vi "playback_choose_freq.vi"() -> ()   [LabVIEW 2012]
doc: "This VI will initialize the FPGA VI and read a user-defined number of samples from a DMA FIFO. When the data acquisition is complete this VI will read status information from the FPGA VI.\n\nFollow these instructions to run the VI.\n\n1. Select your RIO device from the dropdown.\n2. Set the sample period, number of samples to acquire per channel, and DMA block read size. \n\nNote: the block read size should be set to balance load on the host processor and the update rate of the user interface. A small block read size will update the user interface more often but will result in a higher load on the host processor."
uses:
  <vilib>/Analysis/3filter.llb/Filter Passband Type.ctl
  <vilib>/Analysis/3filter.llb/Elliptic Filter (DBL).vi
  <vilib>/Analysis/3filter.llb/Butterworth Filter (DBL).vi
  <vilib>/Analysis/NI_AALBase.lvlib
panel:
  in  "Noise length":i32=50
  out "threshold 0":dbl(graph)
  in  "Filter mode":enum16{"Elliptic", "Butterworth"}(ring)=enum."Butterworth"
  in  "order":i32=3
  in  "low cutoff freq: fl":dbl=20000.0
  in  "high cutoff freq: fh":dbl=30000.0
  out "Selected Index":i32
  out "Ratio at Index (%)":dbl
  in  "Threshold":dbl=0.1
  out "Index 0":dbl
  out "Index 1":dbl
  out "Index 2":dbl
  out "Index 3":dbl
  in  "noise min":dbl=0.001
  out "amplitude 0":dbl
  out "amplitude 1":dbl
  out "amplitude 2":dbl
  out "amplitude 3":dbl
  in  "Portion Duration":i32=600
  in  "Altitude":dbl=2.0
  out "x":dbl format="%#_6f"
  out "y":dbl format="%#_6f"
  out "z":dbl
  out "yaw":dbl
  out "pitch":dbl
  out "Yaw Chart":dbl(graph)
  in  "Mode":T1(ring)=enum."Use Far Field"
  out "Threshold 0":dbl
  out "Threshold 1":dbl
  out "Threshold 2":dbl
  out "Threshold 3":dbl
  in  "threshold ratio":dbl=3.0
  out "bad signal?":bool
  out "ROS  Error":bool
  in  "Send to ROS":bool
  out "dt1":dbl
  out "dt2":dbl
  out "dt3":dbl
  out "Forward":dbl
  out "Sidemove":dbl
  out "Extracted signal":dbl[][](graph)
  in  "Select Frequency":dbl=24000.0
  out "frequency 2":dbl
  out "frequency 1":dbl
  out "Chosen Signal":dbl[][](graph)
  in  "Wait?":bool
  in  "Next Signal":bool
  in  "Filename":path=path "D:/Recorded/US Test/Robosub day 1/pinger_in_front.tdms"
  out "Original Filtered Ch0":dbl[](graph)
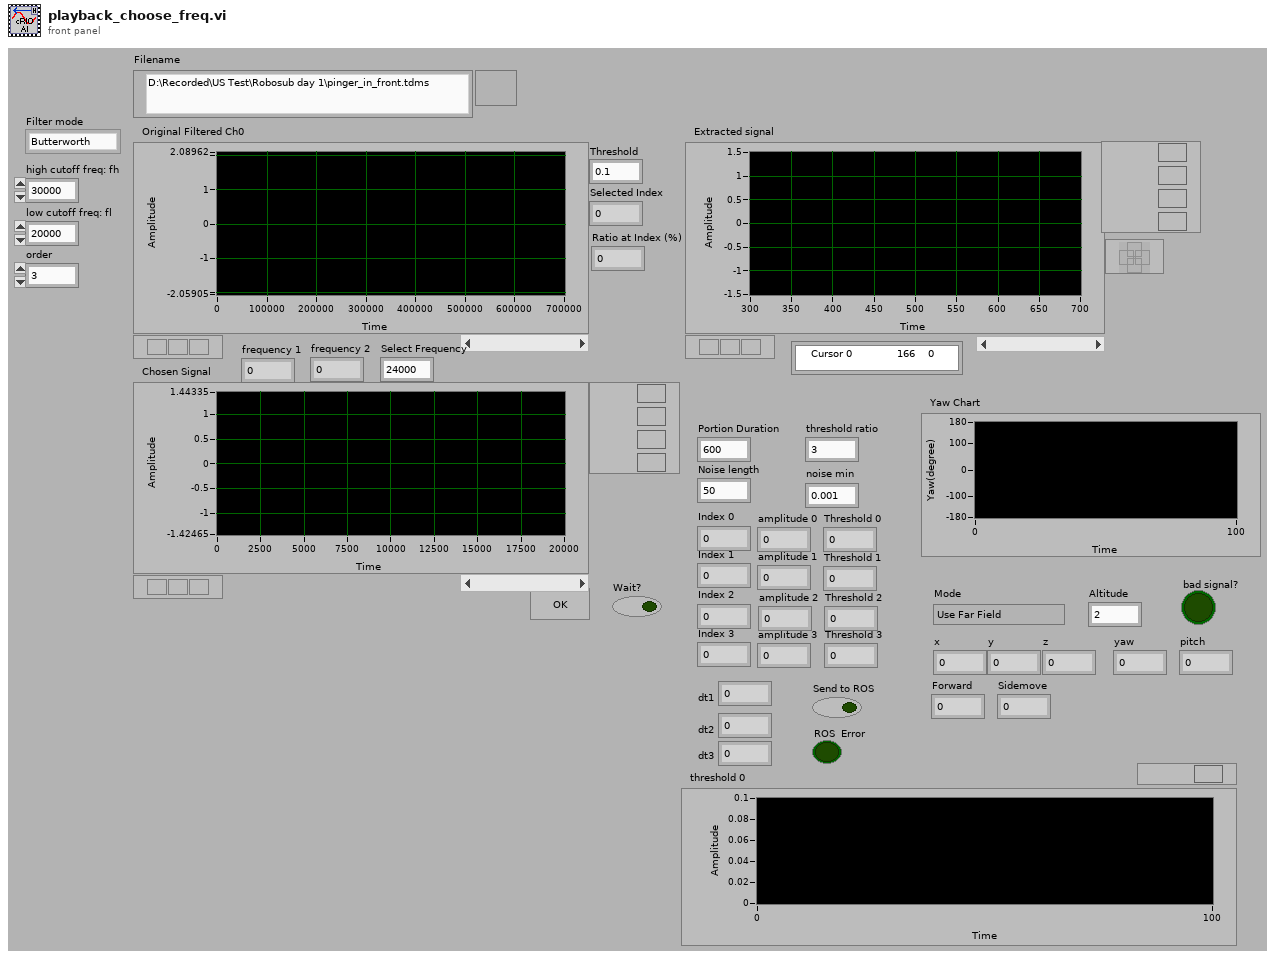
[diagram p1: front panel]
types:
  T1 = enum16{"Use Near Field", "Use Far Field", "Far Field with 3 hydrophones"}
  T2 = typedef "NI_AALBase.lvlib/Filter Passband Type.ctl" = enum32{"Lowpass", "Highpass", "Bandpass", "Bandstop"}
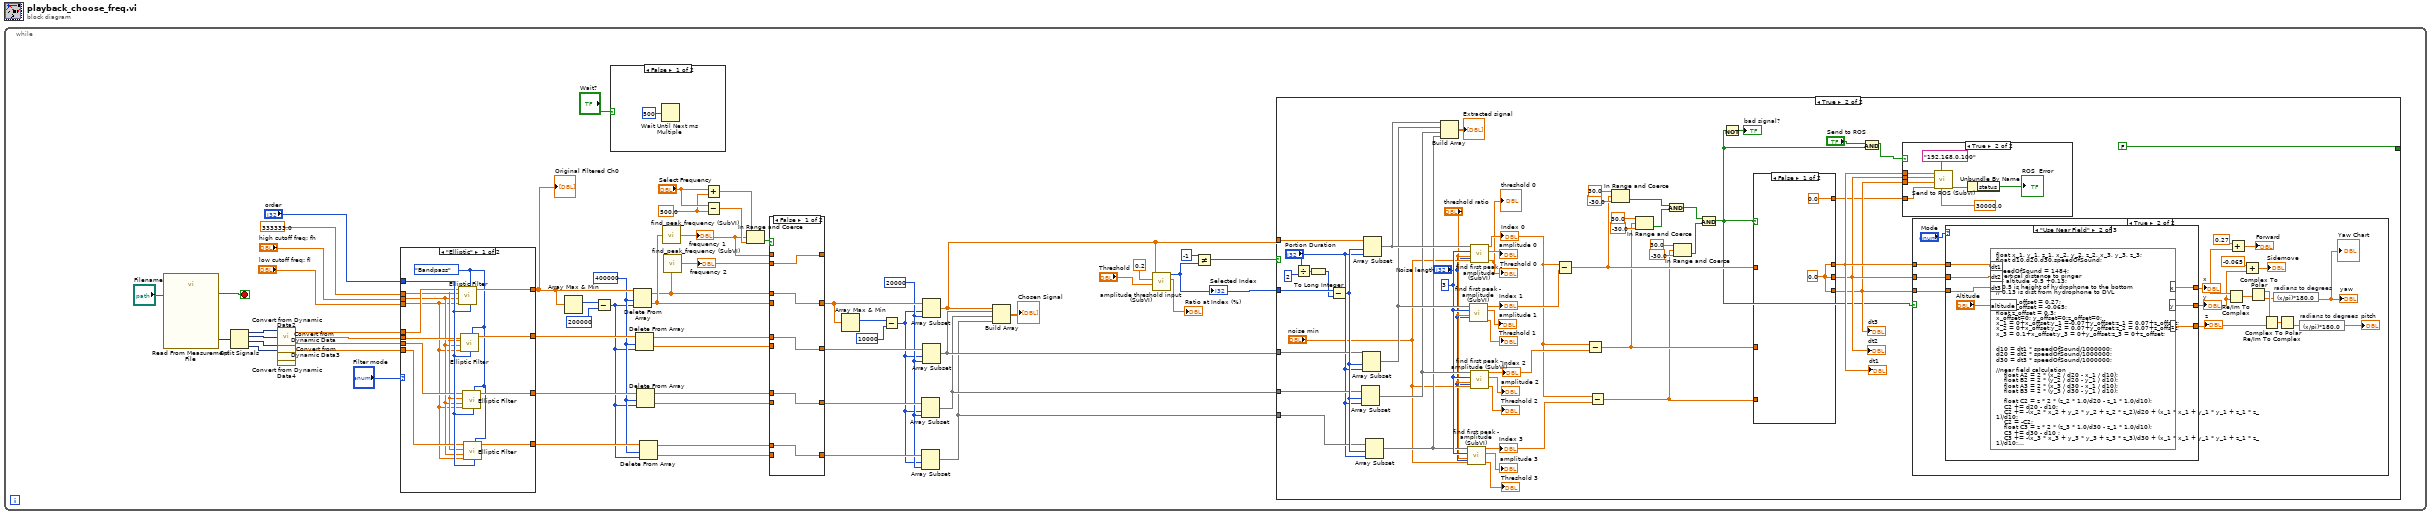
[diagram p0: block diagram]
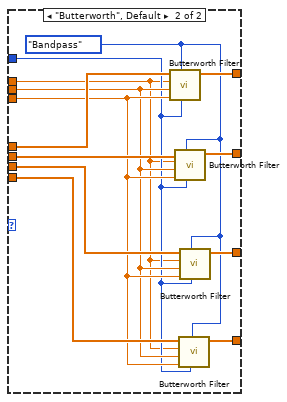
[diagram p2: hidden frame]
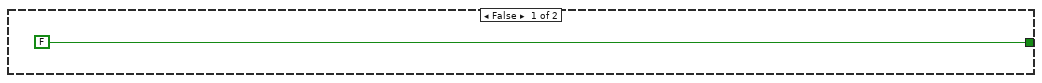
[diagram p3: hidden frame]
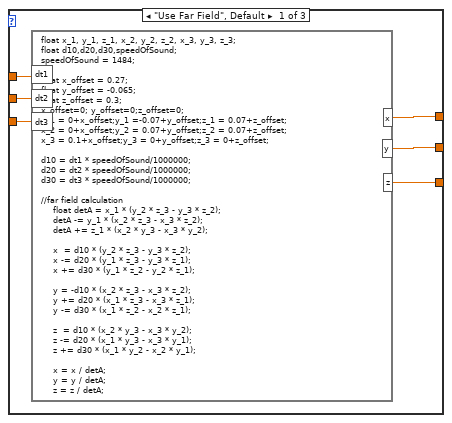
[diagram p5: hidden frame]
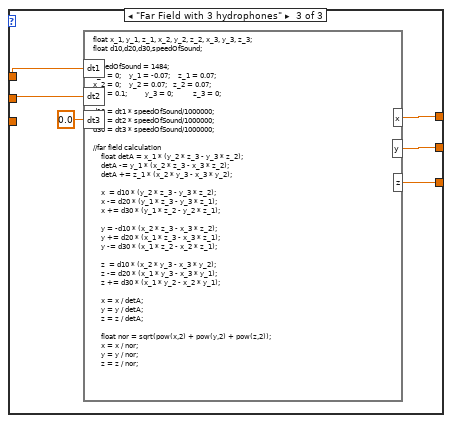
[diagram p6: hidden frame]
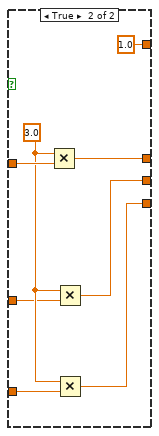
[diagram p8: hidden frame]
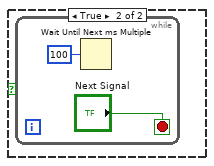
[diagram p9: hidden frame]
diagram:
  n1 = while {
    stop <- w52 stop-if-true
    w23 = 500.0 ("y")
    w29 = 20000 ("length")
    w43 = 400000 ("Portion Duration")
    n2 = call "Read From Measurement File"("Filename"="Filename") -> ("Signals"=w56:dynamicdata, "EOF?"=w52:bool)  [unwired: 5 in, 4 out]
    n3 = Split Signals(w56) -> (w3:dynamicdata, w59:dynamicdata, w58:dynamicdata, w57:dynamicdata)  [unwired: 4 in]
    n4 = call "Convert from Dynamic Data"("Dynamic Data Type"=w3) -> ("Array"=w50:dbl[])  [unwired: 3 in]
    n5 = call "Convert from Dynamic Data2"("Dynamic Data Type"=w59) -> ("Array"=w55:dbl[])  [unwired: 3 in]
    n6 = call "Convert from Dynamic Data3"("Dynamic Data Type"=w58) -> ("Array"=w53:dbl[])  [unwired: 3 in]
    n7 = call "Convert from Dynamic Data4"("Dynamic Data Type"=w57) -> ("Array"=w54:dbl[])  [unwired: 3 in]
    n8 = case shown="\"Elliptic\"" "Filter mode" {
      tunnel: w55 -> [w66 w85]
      tunnel: w54 -> [w64 w84]
      tunnel: w53 -> [w65 w83]
      tunnel: w50 -> [w67 w82]
      tunnel: [w72 w81] -> w49
      tunnel: [w71 w80] -> w46
      tunnel: [w70 w79] -> w45
      tunnel: [w69 w78] -> w44
      tunnel: "low cutoff freq: fl" -> [w60 w77]
      tunnel: "high cutoff freq: fh" -> [w61 w76]
      tunnel: "order" -> [w68 w75]
      tunnel: 333333.0 ("sampling freq: fs") -> [w62 w74]
      frame "Elliptic" {
        w63 = Filter_Passband_Type."Bandpass" ("filter type")
        n9 = call-poly <vilib>:"Elliptic Filter.vi"("order"=w68, "filter type"=w63, "low cutoff freq: fl"=w60, "high cutoff freq: fh"=w61, "sampling freq: fs"=w62, "X"=w67) -> ("Filtered X"=w72:dbl[])  [unwired: 4 in, 1 out]
        n10 = call-poly <vilib>:"Elliptic Filter.vi"("order"=w68, "filter type"=w63, "low cutoff freq: fl"=w60, "high cutoff freq: fh"=w61, "sampling freq: fs"=w62, "X"=w66) -> ("Filtered X"=w71:dbl[])  [unwired: 4 in, 1 out]
        n11 = call-poly <vilib>:"Elliptic Filter.vi"("order"=w68, "filter type"=w63, "low cutoff freq: fl"=w60, "high cutoff freq: fh"=w61, "sampling freq: fs"=w62, "X"=w65) -> ("Filtered X"=w70:dbl[])  [unwired: 4 in, 1 out]
        n12 = call-poly <vilib>:"Elliptic Filter.vi"("order"=w68, "filter type"=w63, "low cutoff freq: fl"=w60, "high cutoff freq: fh"=w61, "sampling freq: fs"=w62, "X"=w64) -> ("Filtered X"=w69:dbl[])  [unwired: 4 in, 1 out]
      }
      frame "Butterworth", Default {
        w73 = Filter_Passband_Type."Bandpass" ("filter type")
        n13 = call-poly <vilib>:"Butterworth Filter.vi"("order"=w75, "filter type"=w73, "low cutoff freq: fl"=w77, "high cutoff freq: fh"=w76, "sampling freq: fs"=w74, "X"=w82) -> ("Filtered X"=w81:dbl[])  [unwired: 2 in, 1 out]
        n14 = call-poly <vilib>:"Butterworth Filter.vi"("order"=w75, "filter type"=w73, "low cutoff freq: fl"=w77, "high cutoff freq: fh"=w76, "sampling freq: fs"=w74, "X"=w85) -> ("Filtered X"=w80:dbl[])  [unwired: 2 in, 1 out]
        n15 = call-poly <vilib>:"Butterworth Filter.vi"("order"=w75, "filter type"=w73, "low cutoff freq: fl"=w77, "high cutoff freq: fh"=w76, "sampling freq: fs"=w74, "X"=w84) -> ("Filtered X"=w78:dbl[])  [unwired: 2 in, 1 out]
        n16 = call-poly <vilib>:"Butterworth Filter.vi"("order"=w75, "filter type"=w73, "low cutoff freq: fl"=w77, "high cutoff freq: fh"=w76, "sampling freq: fs"=w74, "X"=w83) -> ("Filtered X"=w79:dbl[])  [unwired: 2 in, 1 out]
      }
    }
    "Original Filtered Ch0" <- w49
    n17 = Array Max & Min(array=w49) -> (max index (indices)=w48:i32)  [unwired: 3 out]
    n18 = Subtract(x=w48, y=200000) -> (x-y=w42:i32)
    n19 = case shown="False" "Wait?" {
      frame False {
        n20 = Wait Until Next ms Multiple(millisecond multiple=u32 500) -> ()  [unwired: 1 out]
      }
      frame True {
        n21 = while {
          stop <- "Next Signal" stop-if-true
          n22 = Wait Until Next ms Multiple(millisecond multiple=u32 100) -> ()  [unwired: 1 out]
        }
      }
    }
    n23 = Delete From Array(array=w49, length=w43, index=w42) -> (deleted portion=w26:dbl[], array with subset deleted=w25:dbl[])
    n24 = Delete From Array(array=w46, length=w43, index=w42) -> (deleted portion=w41:dbl[], array with subset deleted=w38:dbl[])
    n25 = Delete From Array(array=w45, length=w43, index=w42) -> (deleted portion=w40:dbl[], array with subset deleted=w37:dbl[])
    n26 = Delete From Array(array=w44, length=w43, index=w42) -> (deleted portion=w39:dbl[], array with subset deleted=w36:dbl[])
    n27 = call "find_peak_frequency (SubVI).vi"("Signal"=w26) -> ("Frequency"=w19:dbl)
    "frequency 1" <- w19
    n28 = call "find_peak_frequency (SubVI).vi"("Signal"=w25) -> ("Frequency"=w18:dbl)
    "frequency 2" <- w18
    n29 = Add(x="Select Frequency", y=w23) -> (x+y=w21:dbl)
    n30 = Subtract(x="Select Frequency", y=w23) -> (x-y=w20:dbl)
    n31 = In Range and Coerce(upper limit=w21, x=w19, lower limit=w20) -> (In Range?=w22:bool)  [unwired: 1 out]
    n32 = case shown="False" w22 {
      tunnel: w26 -> [_ w207]
      tunnel: w41 -> [_ w206]
      tunnel: w40 -> [_ w205]
      tunnel: w39 -> [_ w204]
      tunnel: w25 -> [w202 _]
      tunnel: w38 -> [w201 _]
      tunnel: w37 -> [w200 _]
      tunnel: w36 -> [w199 _]
      tunnel: [w202 w207] -> w33
      tunnel: [w201 w206] -> w32
      tunnel: [w200 w205] -> w31
      tunnel: [w199 w204] -> w30
      tunnel: [w198 w203] -> _
      tunnel: w19 -> [_ w203]
      tunnel: w18 -> [w198 _]
      frame False {
      }
      frame True {
      }
    }
    n33 = Array Max & Min(array=w33) -> (max index (indices)=w34:i32)  [unwired: 3 out]
    n34 = Subtract(x=w34, y=10000) -> (x-y=w28:i32)
    n35 = Array Subset(array=w31, index=w28, length=w29) -> (w8:dbl[])
    n36 = Array Subset(array=w30, index=w28, length=w29) -> (w7:dbl[])
    n37 = Array Subset(array=w33, index=w28, length=w29) -> (w10:dbl[])
    n38 = Array Subset(array=w32, index=w28, length=w29) -> (w9:dbl[])
    n39 = Build Array(w10, w9, w8, w7) -> (→"Chosen Signal":dbl[][])
    n40 = call "amplitude threshold input (SubVI).vi"("threshold"="Threshold", "%max amplitude"=0.2, "Array"=w10) -> ("actual ratio (%)"=→"Ratio at Index (%)":dbl, "Index"=w11:i32)  [unwired: 7 in]
    "Selected Index" <- w11
    n41 = Not Equal?(x=-1 ("y"), y=w11) -> (x != y?=w15:bool)
    n42 = case shown="True" w15 {
      tunnel: w9 -> [_ w138]
      tunnel: w8 -> [_ w137]
      tunnel: w7 -> [_ w136]
      tunnel: w10 -> [_ w135]
      tunnel: w11 -> [_ w134]
      tunnel: [FALSE ("Debug") FALSE ("Debug")] -> _
      frame False {
      }
      frame True {
        w100 = 3
        n43 = Divide(x="Portion Duration", y=2) -> (x/y=w131:dbl)
        n44 = To Long Integer(number=w131) -> (32bit integer=w130:i32)
        n45 = Subtract(x=w134, y=w130) -> (x-y=w139:i32)
        n46 = Array Subset(array=w137, index=w139, length="Portion Duration") -> (w101:dbl[])
        n47 = Array Subset(array=w138, index=w139, length="Portion Duration") -> (w105:dbl[])
        n48 = Array Subset(array=w135, index=w139, length="Portion Duration") -> (w107:dbl[])
        n49 = Array Subset(array=w136, index=w139, length="Portion Duration") -> (w99:dbl[])
        n50 = Build Array(w107, w105, w101, w99) -> (→"Extracted signal":dbl[][])
        n51 = call "find first peak - amplitude (SubVI).vi"("Noise duration (units)"="Noise length", "Noise min (amplitude)"="noise min", "threshold ratio"="threshold ratio", "peak width (units)"=w100, "Array"=w99) -> ("Peak threshold"=→"Threshold 3":dbl, "peak amplitude"=→"amplitude 3":dbl, "Index"=w98:dbl)  [unwired: 2 in, 2 out]
        "Index 3" <- w98
        n52 = call "find first peak - amplitude (SubVI).vi"("Noise duration (units)"="Noise length", "threshold ratio"="threshold ratio", "peak width (units)"=w100, "Array"=w105) -> ("Peak threshold"=→"Threshold 1":dbl, "peak amplitude"=→"amplitude 1":dbl, "Index"=w104:dbl)  [unwired: 3 in, 2 out]
        "Index 1" <- w104
        n53 = call "find first peak - amplitude (SubVI).vi"("Noise duration (units)"="Noise length", "Noise min (amplitude)"="noise min", "threshold ratio"="threshold ratio", "peak width (units)"=w100, "Array"=w107) -> ("Peak threshold"=→"Threshold 0" →"threshold 0":dbl, "peak amplitude"=→"amplitude 0":dbl, "Index"=w94:dbl)  [unwired: 2 in, 2 out]
        "Index 0" <- w94
        n54 = call "find first peak - amplitude (SubVI).vi"("Noise duration (units)"="Noise length", "Noise min (amplitude)"="noise min", "threshold ratio"="threshold ratio", "peak width (units)"=w100, "Array"=w101) -> ("Peak threshold"=→"Threshold 2":dbl, "peak amplitude"=→"amplitude 2":dbl, "Index"=w102:dbl)  [unwired: 2 in, 2 out]
        "Index 2" <- w102
        n55 = Subtract(x=w94, y=w104) -> (x-y=w126:dbl)
        n56 = Subtract(x=w94, y=w102) -> (x-y=w123:dbl)
        n57 = Subtract(x=w94, y=w98) -> (x-y=w120:dbl)
        n58 = In Range and Coerce(upper limit=30.0, x=w126, lower limit=-30.0) -> (In Range?=w119:bool)  [unwired: 1 out]
        n59 = In Range and Coerce(upper limit=30.0, x=w123, lower limit=-30.0) -> (In Range?=w118:bool)  [unwired: 1 out]
        n60 = And(x=w119, y=w118) -> (x .and. y?=w117:bool)
        n61 = In Range and Coerce(upper limit=30.0, x=w120, lower limit=-30.0) -> (In Range?=w116:bool)  [unwired: 1 out]
        n62 = And(x=w117, y=w116) -> (x .and. y?=w108:bool)
        n63 = Not(x=w108) -> (.not. x?=→"bad signal?":bool)
        n64 = case shown="False" w108 {
          tunnel: w126 -> [_ w194]
          tunnel: w123 -> [_ w192]
          tunnel: w120 -> [_ w191]
          tunnel: [w185 w190] -> w113
          tunnel: [w185 w189] -> w112
          tunnel: [w185 w188] -> w111
          tunnel: [0.0 ("x") 1.0 ("x")] -> w110
          frame False {
            w185 = 0.0
          }
          frame True {
            w193 = 3.0 ("x")
            n65 = Multiply(x=w193, y=w194) -> (x*y=w190:dbl)
            n66 = Multiply(x=w193, y=w192) -> (x*y=w189:dbl)
            n67 = Multiply(x=w193, y=w191) -> (x*y=w188:dbl)
          }
        }
        "dt1" <- w113
        "dt2" <- w112
        "dt3" <- w111
        n68 = And(x="Send to ROS", y=w108) -> (x .and. y?=w109:bool)
        n69 = case shown="True" w109 {
          tunnel: w113 -> [_ w180]
          tunnel: w112 -> [_ w179]
          tunnel: w111 -> [_ w178]
          tunnel: w110 -> [_ w177]
          frame False {
          }
          frame True {
            n70 = call "Send to ROS (SubVI).vi"("frequency"=30000.0, "ROS IP"="192.168.0.100", "Good signal?"=w177, "dt 3"=w178, "dt2"=w179, "dt 1"=w180) -> ("error out"=w183:errorcluster)  [unwired: 5 in]
            n71 = Unbundle By Name(w183) -> ("status"=→"ROS  Error":bool)
          }
        }
        n72 = case shown="True" w108 {
          tunnel: w113 -> [_ w148]
          tunnel: w112 -> [_ w147]
          tunnel: w111 -> [_ w146]
          frame False {
          }
          frame True {
            n73 = case shown="\"Use Near Field\"" "Mode" {
              tunnel: [w163 w170 w175] -> w145
              tunnel: [w162 w169 w174] -> w142
              tunnel: [w161 w168 w173] -> w152
              tunnel: w148 -> [w160 w166 w172]
              tunnel: w147 -> [w159 w165 w171]
              tunnel: w146 -> [w158 w164 _]
              frame "Use Far Field", Default {
                n74 = formula code="float x_1, y_1, z_1, x_2, y_2, z_2, x_3, y_3, z_3;\nfloat d10,d20,d30,speedOfSound;\nspeedOfSound = 1484;\n\nfloat x_offset = 0.27;\nfloat y_offset = -0.065;\nfloat z_offset = 0.3;\nx_offset=0; y_offset=0;z_offset=0;\nx_1 = 0+x_offset;y_1 =-0.07+y_offset;z_1 = 0.07+z_offset;\nx_2 = 0+x_offset;y_2 = 0.07+y_offset;z_2 = 0.07+z_offset;\nx_3 = 0.1+x_offset;y_3 = 0+y_offset;z_3 = 0+z_offset;\n\nd10 = dt1 * speedOfSound/1000000;\nd20 = dt2 * speedOfSound/1000000;\nd30 = dt3 * speedOfSound/1000000;\n\n//far field calculation\n    float detA = x_1 * (y_2 * z_3 - y_3 * z_2);\n    detA -= y_1 * (x_2 * z_3 - x_3 * z_2);\n    detA += z_1 * (x_2 * y_3 - x_3 * y_2);\n\n    x  = d10 * (y_2 * z_3 - y_3 * z_2);\n    x -= d20 * (y_1 * z_3 - y_3 * z_1);\n    x += d30 * (y_1 * z_2 - y_2 * z_1);\n\n    y = -d10 * (x_2 * z_3 - x_3 * z_2);\n    y += d20 * (x_1 * z_3 - x_3 * z_1);\n    y -= d30 * (x_1 * z_2 - x_2 * z_1);\n\n    z  = d10 * (x_2 * y_3 - x_3 * y_2);\n    z -= d20 * (x_1 * y_3 - x_3 * y_1);\n    z += d30 * (x_1 * y_2 - x_2 * y_1);\n\n    x = x / detA;\n    y = y / detA;\n    z = z / detA;\n\n    float nor = sqrt(pow(x,2) + pow(y,2) + pow(z,2));\n    x = x / nor;\n    y = y / nor;\n    z = z / nor;"("dt1"=w160, "dt2"=w159, "dt3"=w158) -> ("x"=w163:dbl, "y"=w162:dbl, "z"=w161:dbl)
              }
              frame "Use Near Field" {
                n75 = formula code="float x_1, y_1, z_1, x_2, y_2, z_2, x_3, y_3, z_3;\nfloat d10,d20,d30,speedOfSound;\n\nspeedOfSound = 1484;\n//vertical distance to pinger\nz= altitude -0.5 +0.13;\n// 0.5 is height of hydrophone to the bottom\n// 0.13 is dist from hydrophone to DVL\n\nfloat x_offset = 0.27;\nfloat y_offset = -0.065;\nfloat z_offset = 0.3;\nx_offset=0; y_offset=0;z_offset=0;\nx_1 = 0+x_offset;y_1 =-0.07+y_offset;z_1 = 0.07+z_offset;\nx_2 = 0+x_offset;y_2 = 0.07+y_offset;z_2 = 0.07+z_offset;\nx_3 = 0.1+x_offset;y_3 = 0+y_offset;z_3 = 0+z_offset;\n\n\nd10 = dt1 * speedOfSound/1000000;\nd20 = dt2 * speedOfSound/1000000;\nd30 = dt3 * speedOfSound/1000000;\n\n//near field calculation\n    float A2 = 2 * (x_2 / d20 - x_1 / d10);\n    float B2 = 2 * (y_2 / d20 - y_1 / d10);\n    float A3 = 2 * (x_3 / d30 - x_1 / d10);\n    float B3 = 2 * (y_3 / d30 - y_1 / d10);\n    \n    float C2 = z * 2 * (z_2 * 1.0/d20 - z_1 * 1.0/d10);\n    C2 += d20 - d10;\n    C2 += -(x_2 * x_2 + y_2 * y_2 + z_2 * z_2)/d20 + (x_1 * x_1 + y_1 * y_1 + z_1 * z_1)/d10;\n    C2 = -C2;\n    float C3 = z * 2 * (z_3 * 1.0/d30 - z_1 * 1.0/d10);\n    C3 += d30 - d10 ;\n    C3 += -(x_3 * x_3 + y_3 * y_3 + z_3 * z_3)/d30 + (x_1 * x_1 + y_1 * y_1 + z_1 * z_1)/d10;\n    C3 = -C3;\n\n    if (A2*B3 == A3*B2) {\n        x = 0;\n        y = 0;\n    }\n    else {\n        x = (C2 * B3 - C3 * B2) / (A2 * B3 - A3 * B2);\n        y = (C3 * A2 - C2 * A3) / (B3 * A2 - B2 * A3);\n    }"("dt1"=w166, "dt2"=w165, "dt3"=w164, "altitude"="Altitude") -> ("x"=w170:dbl, "y"=w169:dbl, "z"=w168:dbl)
              }
              frame "Far Field with 3 hydrophones" {
                n76 = formula code="float x_1, y_1, z_1, x_2, y_2, z_2, x_3, y_3, z_3;\nfloat d10,d20,d30,speedOfSound;\n\nspeedOfSound = 1484;\nx_1 = 0;    y_1 = -0.07;    z_1 = 0.07;\nx_2 = 0;    y_2 = 0.07;   z_2 = 0.07;\nx_3 = 0.1;         y_3 = 0;          z_3 = 0;\n\nd10 = dt1 * speedOfSound/1000000;\nd20 = dt2 * speedOfSound/1000000;\nd30 = dt3 * speedOfSound/1000000;\n\n//far field calculation\n    float detA = x_1 * (y_2 * z_3 - y_3 * z_2);\n    detA -= y_1 * (x_2 * z_3 - x_3 * z_2);\n    detA += z_1 * (x_2 * y_3 - x_3 * y_2);\n\n    x  = d10 * (y_2 * z_3 - y_3 * z_2);\n    x -= d20 * (y_1 * z_3 - y_3 * z_1);\n    x += d30 * (y_1 * z_2 - y_2 * z_1);\n\n    y = -d10 * (x_2 * z_3 - x_3 * z_2);\n    y += d20 * (x_1 * z_3 - x_3 * z_1);\n    y -= d30 * (x_1 * z_2 - x_2 * z_1);\n\n    z  = d10 * (x_2 * y_3 - x_3 * y_2);\n    z -= d20 * (x_1 * y_3 - x_3 * y_1);\n    z += d30 * (x_1 * y_2 - x_2 * y_1);\n\n    x = x / detA;\n    y = y / detA;\n    z = z / detA;\n\n    float nor = sqrt(pow(x,2) + pow(y,2) + pow(z,2));\n    x = x / nor;\n    y = y / nor;\n    z = z / nor;"("dt1"=w172, "dt2"=w171, "dt3"=0.0 ("input variable")) -> ("x"=w175:dbl, "y"=w174:dbl, "z"=w173:dbl)
              }
            }
            "x" <- w145
            "y" <- w142
            "z" <- w152
            n77 = Re/Im To Complex(1:w142, 2:w145) -> (0:w150:cdb)
            n78 = Add(x=0.27, y=w145) -> (x+y=→"Forward":dbl)
            n79 = Add(x=-0.065, y=w142) -> (x+y=→"Sidemove":dbl)
            n80 = Complex To Polar(r * e^(i*theta)=w150) -> (r=w153:dbl, theta=w151:dbl)
            n81 = Re/Im To Complex(1:w152, 2:w153) -> (0:w154:cdb)
            n82 = expression code="(x/pi)*180.0" "radians to degrees"(w151) -> (→"yaw" →"Yaw Chart":dbl)
            n83 = Complex To Polar(r * e^(i*theta)=w154) -> (theta=w156:dbl)  [unwired: 1 out]
            n84 = expression code="(x/pi)*180.0" "radians to degrees"(w156) -> (→"pitch":dbl)
          }
        }
      }
    }
  }
